vi "Continuous Pulse Train Test.vi"() -> ()   [LabVIEW 2015]
uses:
  Waveform VIs/Pulse Train VIs/Pulse Train Params.ctl
  Waveform VIs/Pulse Train VIs/Pulse Polarity.ctl
  Waveform VIs/Pulse Train VIs/PT-Continuous State.ctl
panel:
  out "Numeric":i32
  in  "Phase (cycles)":dbl(slide)=1.0 min=0.0 max=2.0 scale=0.0..2.0
  in  "Pulse Train Params":T1={"Pulse width (us)"=1000.0, "Pulse rate (Hz)"=0.0, "Gap (ms)"=0.0, "Polarity"=enum."POS", "PT State"={"Template"=[], "Nperiod"=0, "Index"=0, "Pulse Rate (Hz)"=0.0, "Phase (cycles)"=0.0, "Noff"=0}, "Asynch"=FALSE}
  out "Graph":dbl[][](graph)
  in  "Buffer (ms)":dbl=50.0
  in  "Pulse Rate (Hz)":dbl(slide)=36.55555555555556 min=1.0 max=100.0 scale=1.0..100.0
  in  "Fs (Hz)":dbl=100000.0
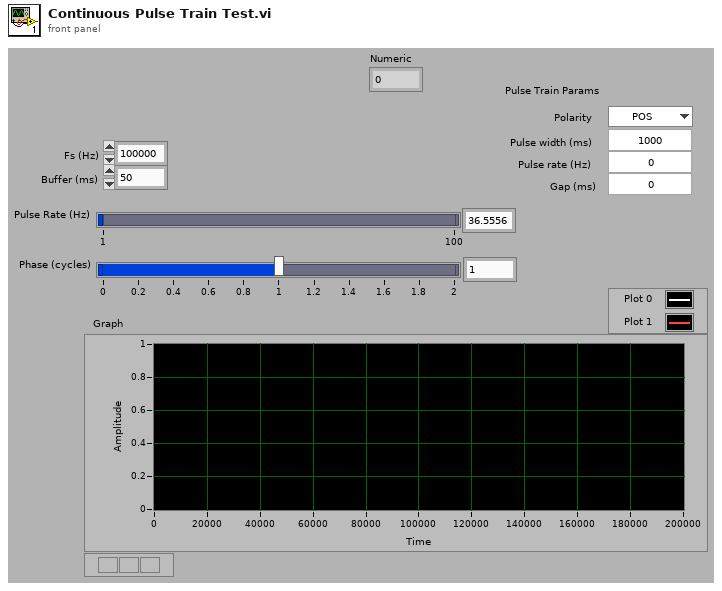
[diagram p1: front panel]
types:
  T1 = typedef "Pulse Train Params.ctl" = cluster{"Pulse width (us)":dbl, "Pulse rate (Hz)":dbl, "Gap (ms)":dbl, "Polarity":T2, "PT State":T3, "Asynch":bool}
  T2 = typedef "Pulse Polarity.ctl" = enum16{"POS", "NEG", "POS-NEG", "NEG-POS"}
  T3 = typedef "PT-Continuous State.ctl" = cluster{"Template":dbl[], "Nperiod":i32, "Index":i32, "Pulse Rate (Hz)":dbl, "Phase (cycles)":dbl, "Noff":i32}
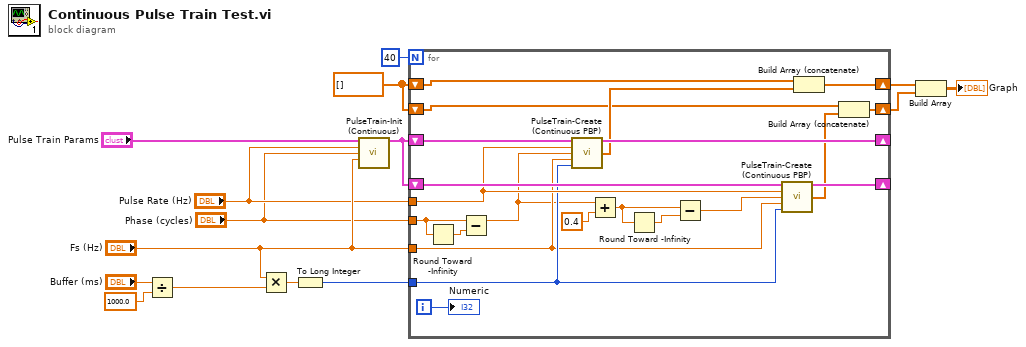
[diagram p0: block diagram]
diagram:
  w6 = dbl[] []
  n1 = Divide(x="Buffer (ms)", y=1000.0) -> (x/y=w13:dbl)
  n2 = Multiply(x="Fs (Hz)", y=w13) -> (x*y=w12:dbl)
  n3 = To Long Integer(number=w12) -> (32bit integer=w10:i32)
  n4 = call "PulseTrain-Init (Continuous).vi"("Pulse Train Params"="Pulse Train Params", "Start Pulse Rate (Hz)"="Pulse Rate (Hz)", "Start Phase (cycles)"="Phase (cycles)", "Fs (Hz)"="Fs (Hz)") -> ("Initial State"=w7:T3)  [unwired: 10 in, 1 out]
  n5 = for {
    N: 40 -> [_]
    tunnel: w10 -> [w28]
    tunnel: "Fs (Hz)" -> [w23]
    shift-right: [w35] -> _
    shift-left: w7 -> [w36]
    shift-right: [w33] -> w5
    shift-left: w6 -> [w32]
    tunnel: "Pulse Rate (Hz)" -> [w29]
    tunnel: "Phase (cycles)" -> [w16]
    shift-right: [w31] -> _
    shift-left: w7 -> [w30]
    shift-right: [w25] -> w4
    shift-left: w6 -> [w24]
    i -> [w20]
    n6 = Round Toward -Infinity(1:w16) -> (0:w17:dbl)
    n7 = Subtract(x=w16, y=w17) -> (x-y=w18:dbl)
    n8 = call "PulseTrain-Create (Continuous PBP).vi"("State In"=w36, "Pulse Rate (Hz)"=w29, "Phase (cycles)"=w18, "Fs (Hz)"=w23, "Npts"=w28) -> ("State Out"=w35:T3, "Buffer"=w34:dbl[])  [unwired: 8 in, 1 out]
    n9 = Add(x=w18, y=0.4) -> (x+y=w21:dbl)
    n10 = Round Toward -Infinity(1:w21) -> (0:w19:dbl)
    n11 = Subtract(x=w21, y=w19) -> (x-y=w22:dbl)
    n12 = call "PulseTrain-Create (Continuous PBP).vi"("State In"=w30, "Pulse Rate (Hz)"=w29, "Phase (cycles)"=w22, "Fs (Hz)"=w23, "Npts"=w28) -> ("State Out"=w31:T3, "Buffer"=w26:dbl[])  [unwired: 8 in, 1 out]
    n13 = Build Array (concatenate)(w32, w34) -> (w33:dbl[])
    n14 = Build Array (concatenate)(w24, w26) -> (w25:dbl[])
    "Numeric" <- w20
  }
  n15 = Build Array(w5, w4) -> (→"Graph":dbl[][])
